vi "InitializePhotoDetector.vi"(9 "error in (no error)":errorcluster {"code" format="%.0x"}, 11 "resource name":refnum<visa-resource-name>) -> (0 "error IO":errorcluster, 3 "instrument handle out":refnum<visa-resource-name>, 5 "Initialized PD":bool)   [LabVIEW 2018]
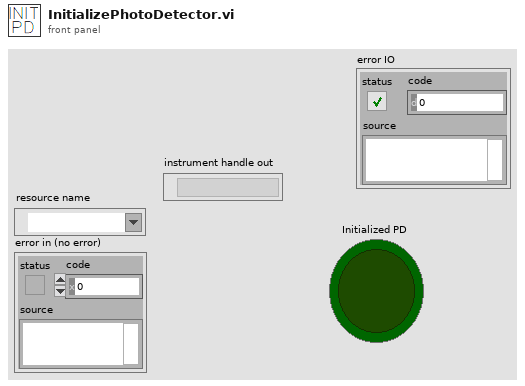
[diagram p1: front panel]
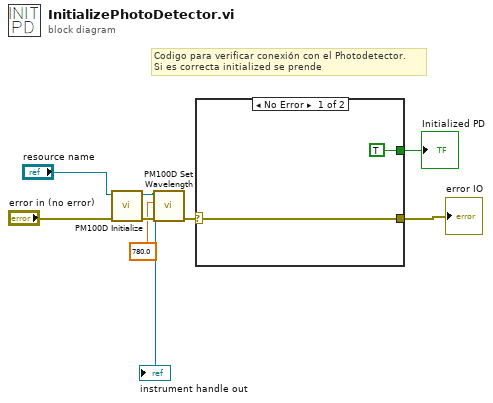
[diagram p0: block diagram]
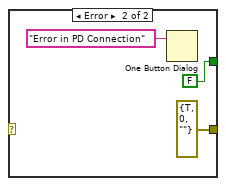
[diagram p2: hidden frame]
diagram:
  # "Codigo para verificar conexión con el Photodetector.\nSi es correcta initialized se prende"
  n1 = call "PM100D Initialize.vi"("error in (no error)"="error in (no error)", "resource name"="resource name") -> ("error out"=w5:errorcluster, "instrument handle out"=w6:refnum<visa-resource-name>)  [unwired: 8 in]
  "instrument handle out" <- w6
  n2 = call "PM100D Set Wavelength.vi"("error in (no error)"=w5, "Wavelength (0.0)"=780.0, "instrument handle"=w6) -> ("error out"=w4:errorcluster)  [unwired: 7 in, 1 out]
  n3 = case shown="No Error" w4 {
    selector: w4 -> [w10 _]
    tunnel: [w10 errorcluster {"status"=TRUE, "code"=0, "source"=""} ("error IO")] -> w1
    tunnel: [TRUE FALSE ("Initialized PD")] -> w3
    frame No Error {
    }
    frame Error {
      n4 = One Button Dialog(message="Error in PD Connection") -> ()  [unwired: 1 in, 1 out]
    }
  }
  "Initialized PD" <- w3
  "error IO" <- w1
